vi "SUB_COM1_SetBootloader_mode.vi"(3 "TimeOut Secs":dbl, 4 "VISA resource name":refnum<visa-resource-name>, 5 "Begin Tick":u32) -> (0 "Output String":string, 2 "Found Bootloader mode":bool)   [LabVIEW 2011]
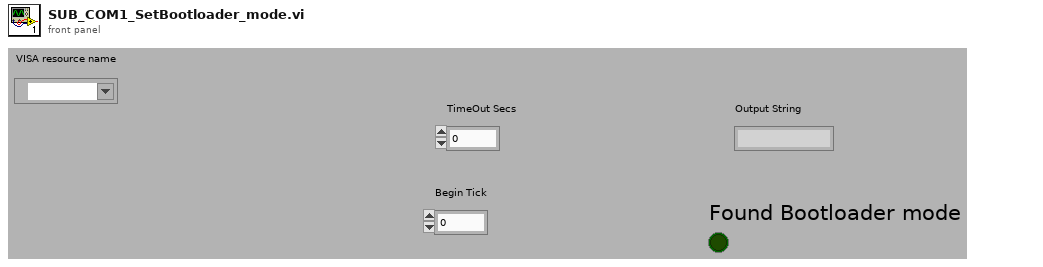
[diagram p1: front panel]
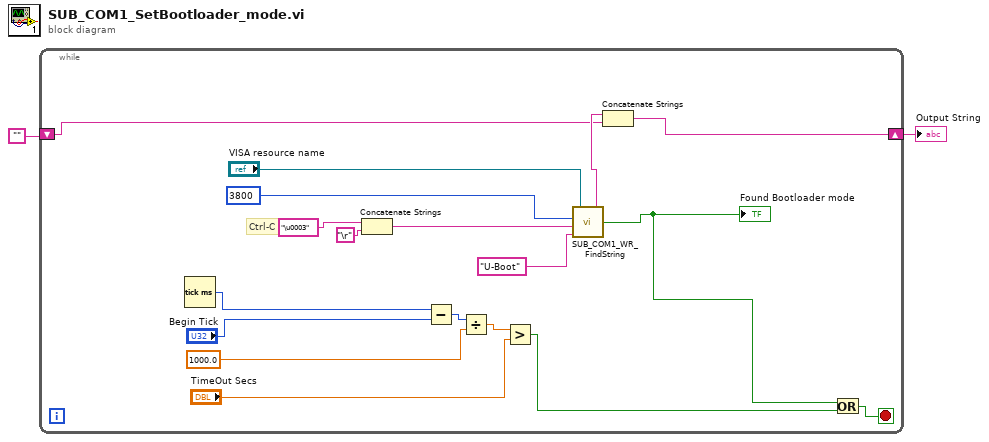
[diagram p0: block diagram]
diagram:
  n1 = while {
    shift-right: [w8] -> w1
    shift-left: "" -> [w7]
    stop <- w14 stop-if-true
    # "Ctrl-C"
    n2 = Tick Count (ms)() -> (millisecond timer value=w18:u32)
    n3 = Concatenate Strings("\u0003" ("write buffer"), "\r") -> (w3:string)
    n4 = Subtract(x=w18, y="Begin Tick") -> (x-y=w17:u32)
    n5 = Divide(x=w17, y=1000.0) -> (x/y=w15:dbl)
    n6 = Greater?(x=w15, y="TimeOut Secs") -> (0:w12:bool)
    n7 = call "SUB_COM1_WR_FindString.vi"("Find this String"="U-Boot", "write buffer"=w3, "number of char to read"=3800, "VISA resource name"="VISA resource name") -> ("Found"=w13:bool, "Output String"=w9:string)  [unwired: 1 out]
    "Found Bootloader mode" <- w13
    n8 = Concatenate Strings(w9, w7) -> (w8:string)
    n9 = Or(x=w13, y=w12) -> (x .or. y?=w14:bool)
  }
  "Output String" <- w1
